vi "getSheetDim.vi"(8 "error in (no error)":errorcluster, 10 "Refnum Cluster Out":T1, 11 "reference in":refnum<class "excelFile.lvclass">) -> (0 "error out":errorcluster, 1 "columnNumber":i32, 2 "rowNumber":i32, 3 "reference out":refnum<class "excelFile.lvclass">)   [LabVIEW 2016, in "excelFile.lvclass"]
uses:
  excelFile.lvclass
  <userlib>/Read_Excel_Values.llb/GetXL_CellValues_2D_String.vi
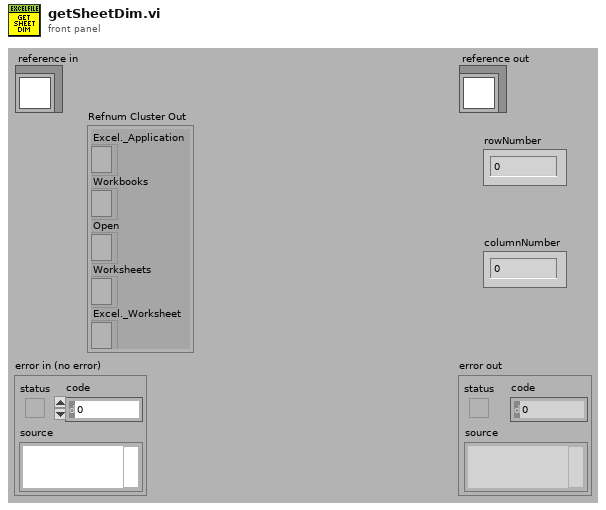
[diagram p1: front panel]
types:
  T1 = cluster{"Excel._Application":refnum<k7>, "Workbooks":refnum<k7>, "Open":refnum<k7>, "Worksheets":refnum<k7>, "Excel._Worksheet":refnum<k7>}
  T2 = typedef "excelFile.lvclass/ObjectAttributesRef.ctl" = refnum<data-value>
  T3 = typedef "excelFile.lvclass/ObjectAttributes.ctl" = cluster{"MyAttribute":dbl, "path":string, "Refnum Excel":cluster{"Excel._Application":refnum<k7>, "Workbooks":refnum<k7>, "Open":refnum<k7>}, "data":string[][][], "save":bool, "fileType":T4, "rowsColor":u32[], "python_ref":refnum<class "python.lvclass">, "items_rows":i32[], "excel_range":i32[][], "TSR":cluster{"number":string, "TSR_path":path, "service_path":path, "email_to":string}, "excel_already_opened?":bool, "file_already_opened?":bool, "excel_protected_opened?":bool, "Refnum Cluster Worksheets":cluster{"Excel._Application":refnum<k7>, "Workbooks":refnum<k7>, "Open":refnum<k7>, "Worksheets":refnum<k7>, "Excel._Worksheet":refnum<k7>}, "#_rows":i32}
  T4 = typedef "excelFile.lvclass/fileType.ctl" = enum16{"devices", "items", "partsTracking", "TSR"}
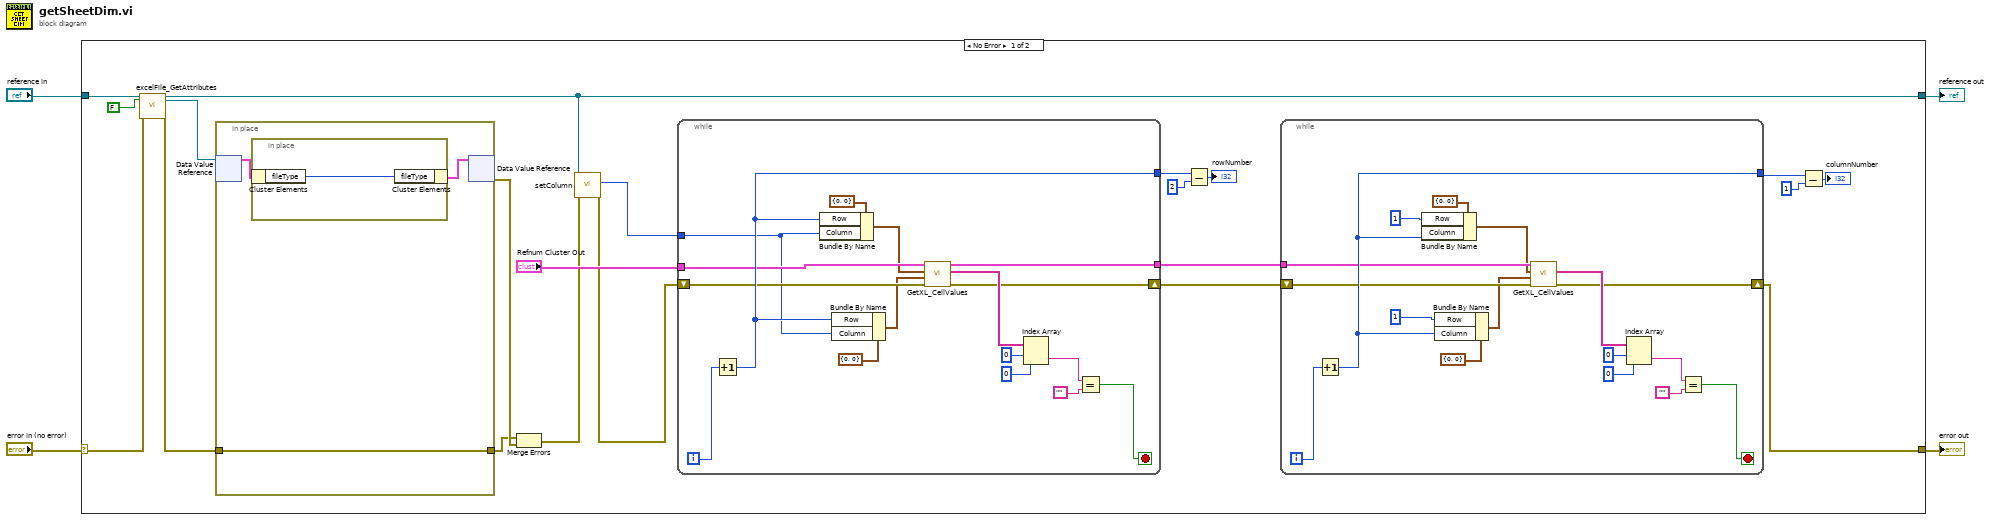
[diagram p0: block diagram]
diagram:
  n1 = case shown="No Error" "error in (no error)" {
    selector: "error in (no error)" -> [w21 w65]
    tunnel: [w12 w65] -> w3
    tunnel: [w7 w64] -> w1
    tunnel: "reference in" -> [w23 w64]
    frame No Error {
      n2 = call "excelFile_GetAttributes.vi"("reference in"=w23, "return data? (T)"=FALSE, "error in (no error)"=w21) -> ("reference out"=w7:refnum<class "excelFile.lvclass">, "attributes ref"=w19:T2, "error out"=w20:errorcluster)  [unwired: 13 in, 1 out]
      n3 = in-place {
        in-place-border: w20 -> [w60]
        in-place-border: [w60] -> w24
        n4 = in-place-dvr #1(w19) -> (w61:T3)  [unwired: 1 out]
        n5 = in-place {
          n6 = in-place-cluster #2(w61) -> ("fileType"=w63:T4)
          n7 = in-place-cluster #2("fileType"=w63) -> (w62:T3)
        }
        n8 = in-place-dvr #1(w62) -> (w25:errorcluster)  [unwired: 1 out]
      }
      n9 = Merge Errors(w24, w25) -> (w6:errorcluster)
      n10 = call "setColumn.vi"("error in (no error)"=w6, "reference in"=w7) -> ("error out"=w5:errorcluster, "column"=w8:i32)  [unwired: 7 in, 1 out]
      n11 = while {
        tunnel: [w46] -> w15
        shift-right: [w44] -> w14
        shift-left: w5 -> [w49]
        tunnel: [w51] -> w17
        tunnel: "Refnum Cluster Out" -> [w50]
        tunnel: w8 -> [w43]
        i -> [w52]
        stop <- w53 stop-if-true
        n12 = Increment(x=w52) -> (x+1=w51:i32)
        n13 = Bundle By Name(cluster=cluster{"Column":i32, "Row":i32} {"Column"=0, "Row"=0} ("Start"), "Row"=w51, "Column"=w43) -> (w48:cluster{"Column":i32, "Row":i32})
        n14 = Bundle By Name(cluster=cluster{"Column":i32, "Row":i32} {"Column"=0, "Row"=0} ("End"), "Row"=w51, "Column"=w43) -> (w47:cluster{"Column":i32, "Row":i32})
        n15 = call-poly <userlib>:"GetXL_CellValues.vi"("error in"=w49, "End"=w47, "Start"=w48, "Refnum Cluster In"=w50) -> ("error out"=w44:errorcluster, "data"=w45:string[][], "Refnum Cluster Out"=w46:T1)  [unwired: 5 in]
        n16 = Index Array(array=w45, index (row)=0, index (col)=0 ("disabled index (col)")) -> (element=w54:string)
        n17 = Equal?(x=w54, y="") -> (x = y?=w53:bool)
      }
      n18 = Subtract(x=w17, y=2) -> (x-y=→"rowNumber":i32)
      n19 = while {
        tunnel: w15 -> [w31]
        shift-right: [w26] -> w12
        shift-left: w14 -> [w30]
        tunnel: [w32] -> w10
        i -> [w35]
        stop <- w36 stop-if-true
        n20 = Increment(x=w35) -> (x+1=w32:i32)
        n21 = Bundle By Name(cluster=cluster{"Column":i32, "Row":i32} {"Column"=0, "Row"=0} ("Start"), "Row"=1 ("Column"), "Column"=w32) -> (w28:cluster{"Column":i32, "Row":i32})
        n22 = Bundle By Name(cluster=cluster{"Column":i32, "Row":i32} {"Column"=0, "Row"=0} ("End"), "Row"=1 ("Column"), "Column"=w32) -> (w29:cluster{"Column":i32, "Row":i32})
        n23 = call-poly <userlib>:"GetXL_CellValues.vi"("error in"=w30, "End"=w29, "Start"=w28, "Refnum Cluster In"=w31) -> ("error out"=w26:errorcluster, "data"=w27:string[][])  [unwired: 5 in, 1 out]
        n24 = Index Array(array=w27, index (row)=0, index (col)=0 ("disabled index (col)")) -> (element=w37:string)
        n25 = Equal?(x=w37, y="") -> (x = y?=w36:bool)
      }
      n26 = Subtract(x=w10, y=1) -> (x-y=→"columnNumber":i32)
    }
    frame Error {
    }
  }
  "error out" <- w3
  "reference out" <- w1
